vi "MongoDB.RenameCollection.vi"(8 "error in (no error)":errorcluster, 9 "newCollectionName":string, 10 "oldCollectionName":string, 11 "MongoDB.Database in":refnum<class "MongoDB.Database.lvclass">) -> (0 "error out":errorcluster, 3 "MongoDB.Database out":refnum<class "MongoDB.Database.lvclass">)   [LabVIEW 2014, in "MongoDB.Database.lvclass"]
uses:
  MongoDB.Database.lvclass
  MongoDB.Database.lvclass/MongoDB.Database.ctl
  C:/Users/Richard/Documents/GitHub/mongo-labview-driver/CSharp/bin/MongoDB.Driver.Legacy.dll
  CSharp/bin/MongoDB.Driver.Legacy.dll
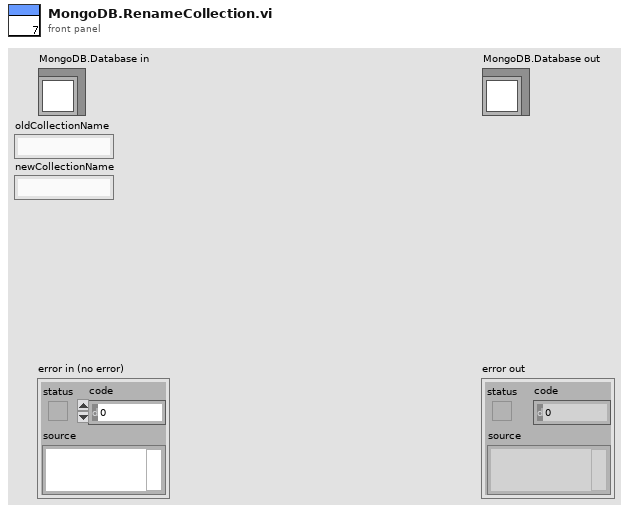
[diagram p1: front panel]
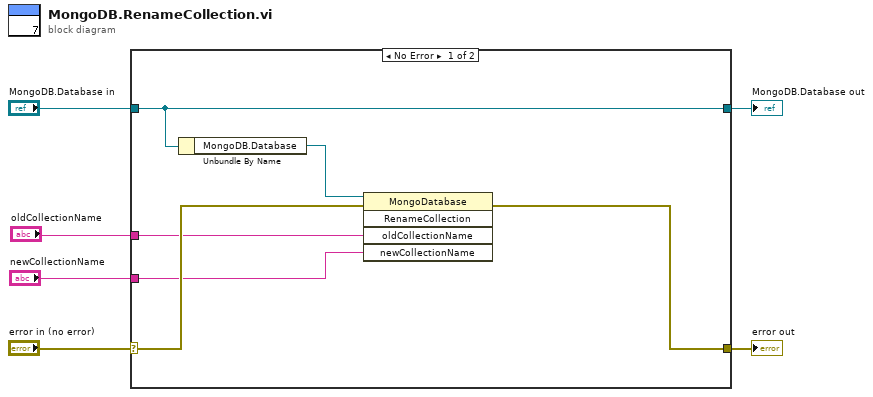
[diagram p0: block diagram]
diagram:
  n1 = case shown="No Error" "error in (no error)" {
    selector: "error in (no error)" -> [w10 w14]
    tunnel: [w9 w14] -> w5
    tunnel: [w12 w13] -> w3
    tunnel: "MongoDB.Database in" -> [w12 w13]
    tunnel: "oldCollectionName" -> [w8 _]
    tunnel: "newCollectionName" -> [w7 _]
    frame No Error {
      n2 = Unbundle By Name(w12) -> ("MongoDB.Database"=w11:refnum<k24>)
      n3 = invoke class="MongoDatabase" method="RenameCollection"(reference=w11, error in=w10, "oldCollectionName"=w8, "newCollectionName"=w7) -> (error out=w9:errorcluster)  [unwired: 1 in, 4 out]
    }
    frame Error {
    }
  }
  "error out" <- w5
  "MongoDB.Database out" <- w3
